vi "Get Framework.vi"(8 "error in (no error)":errorcluster) -> (0 "error out":errorcluster, 2 "Test Framework":refnum<class "Test Framework.lvclass">)   [LabVIEW 2017, in "Framework.lvlib" / "Test Framework Factory.lvclass"]
doc: "Determines the test framework, either from the global configuration or by scanning the application domain."
uses:
  Test Framework Factory.lvclass
  Test Framework/Test Framework.lvclass
  LVUnit Test Framework/LVUnit Test Framework.lvclass
  C:/Users/pasca/Projects/Home/lvunit/Framework/Test Framework/Test Framework.lvclass
  Configuration/Global Configuration/Global Configuration.lvlib
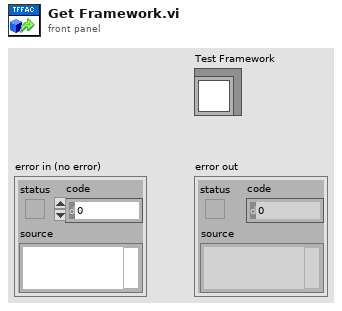
[diagram p1: front panel]
types:
  T1 = typedef "Framework.lvlib/Test Framework.ctl" = enum16{"Unknown", "LVUnit"}
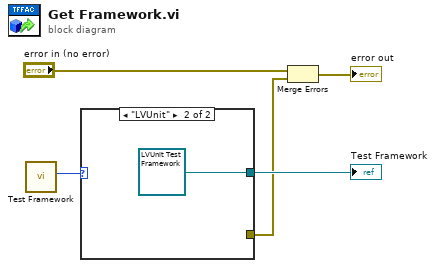
[diagram p0: block diagram]
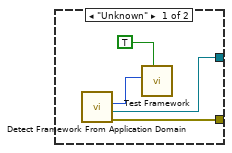
[diagram p2: hidden frame]
diagram:
  n1 = call "Test Framework.vi"() -> ("Test Framework out"=w1:T1)  [unwired: 11 in]
  n2 = case shown="\"LVUnit\"" w1 {
    tunnel: [w8 refnum<class "LVUnit Test Framework.lvclass"> refnum ("Framework.lvlib:LVUnit Test Framework.lvclass")] -> w5
    tunnel: [w9 _] -> w2
    frame "Unknown" {
      n3 = call "Detect Framework From Application Domain.vi"() -> ("error out"=w9:errorcluster, "Test Framework Instance"=w8:refnum<class "Test Framework.lvclass">, "Test Framework Type"=w7:T1)  [unwired: 9 in]
      n4 = call "Test Framework.vi"("Write (F)"=TRUE, "Test Framework (Unknown)"=w7) -> ()  [unwired: 9 in, 1 out]
    }
    frame "LVUnit" {
    }
  }
  "Test Framework" <- w5
  n5 = Merge Errors("error in (no error)", w2) -> (→"error out":errorcluster)
